vi "Test_BooleanTextBinding_ValueOK.vi"(8 "error in (no error)":errorcluster, 11 "TestCase in":refnum<class "TestTransport.lvclass">) -> (0 "error out":errorcluster, 3 "TestCase out":refnum<class "TestTransport.lvclass">)   [LabVIEW 2015, in "Transport.lvlib" / "TestTransport.lvclass"]
uses:
  TestTransport.lvclass
  BooleanTextBinding/BooleanTextBinding.lvclass/BooleanTextBinding.ctl
  BooleanTextBinding/BooleanTextBinding.lvclass
panel:
  out "Button":bool
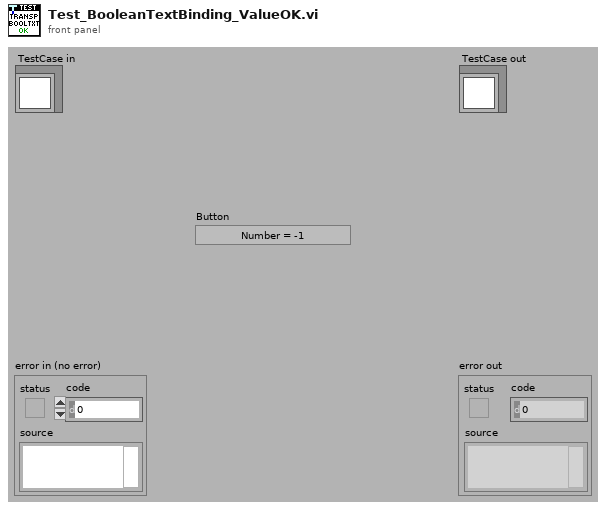
[diagram p1: front panel]
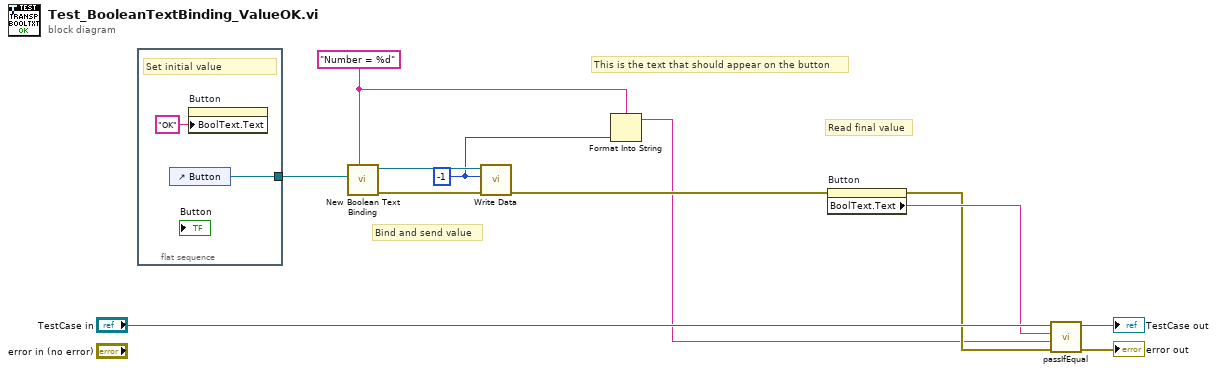
[diagram p0: block diagram]
diagram:
  w3 = "Number = %d" ("Format String")
  w2 = -1
  # "This is the text that should appear on the button"
  # "Bind and send value"
  # "Read final value"
  n1 = flat-sequence {
    tunnel: [w14] -> w6
    frame #0 {
      # "Set initial value"
      n2 = control-ref of="Button"() -> (w14:refnum<vi>)
      n3 = property on="Button" class="Bool"("BoolText.Text"="OK" ("Boolean Text.Text")) -> ()  [unwired: 2 in, 2 out]
    }
  }
  n4 = call "New Boolean Text Binding.vi"("Format String"=w3, "Bool Refnum"=w6) -> ("error out"=w5:errorcluster, "BooleanTextBinding"=w8:refnum<class "BooleanTextBinding.lvclass">)  [unwired: 8 in]
  n5 = call-dynamic "Write Data.vi"("error in (no error)"=w5, "Value"=w2, "BooleanTextBinding in"=w8) -> ("error out"=w7:errorcluster)  [unwired: 7 in, 1 out]
  n6 = Format Into String(format string=w3, w2) -> (resulting string=w1:string)  [unwired: 2 in, 1 out]
  n7 = property on="Button" class="Bool"(error in=w7) -> (error out=w4:errorcluster, "BoolText.Text"=w9:string)  [unwired: 1 in, 1 out]
  n8 = call-dynamic "passIfEqual.vi"("error in (no error)"=w4, "y"=w1, "x"=w9, "TestCase in"="TestCase in") -> ("error out"=→"error out":errorcluster, "TestCase out"=→"TestCase out":refnum<class "TestTransport.lvclass">)  [unwired: 6 in]
